vi "TOBECORRECTEDDeviceDiscover.vi"(0 "GenericDevice in":refnum<class "GenericDevice.lvclass">, 5 "error in (no error)":errorcluster) -> (14 "GenericDevice out":refnum<class "GenericDevice.lvclass">, 15 "results-JSON string":string, 16 "ID":i32, 17 "returned command":string, 18 "error string (if existing)":string, 19 "error out":errorcluster)   [LabVIEW 2023, in "GenericDevice.lvclass"]
uses:
  GenericDevice.lvclass
  GenericDevice.lvclass/GenericDevice.ctl
  f3c4c4a7-1197-4301-b128-d95ffad61759.vi
  8dcdfc4e-e41c-41c3-8bf5-06d7d5a87ca3.vi
  <vilib>/JDP Science/JSONtext/Variant to JSON Text.vi
  <vilib>/JDP Science/JSONtext/Set Item.vi
  <vilib>/JDP Science/JSONtext/LVClass Serializer/JSONtext LVClass Serializer.lvclass
panel:
  # "Connector Pane"
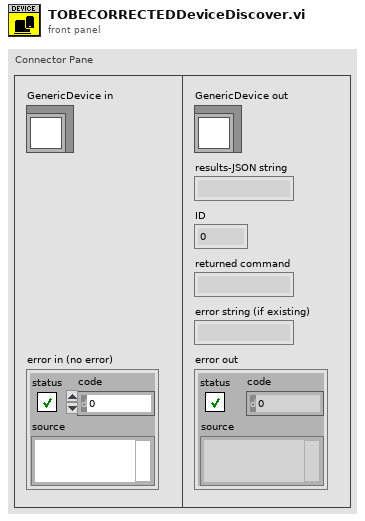
[diagram p1: front panel]
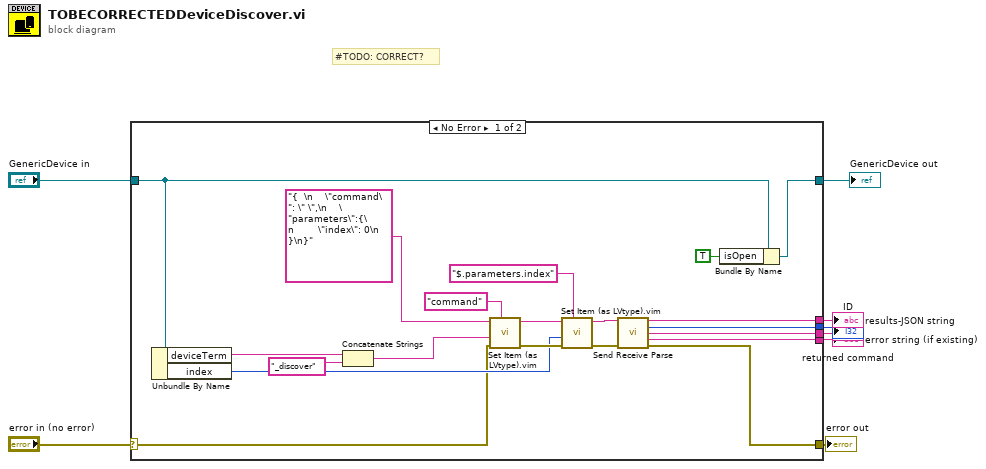
[diagram p0: block diagram]
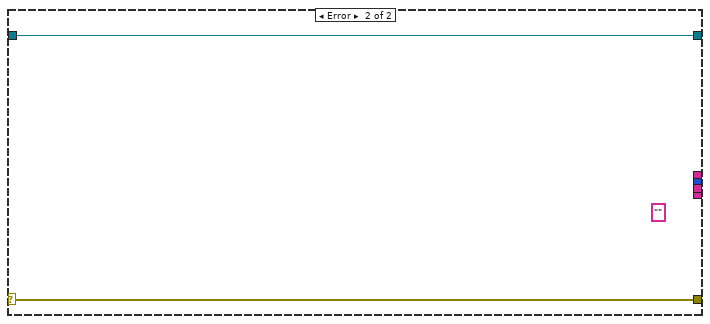
[diagram p2: hidden frame]
diagram:
  # "#TODO: CORRECT?"
  n1 = case shown="No Error" "error in (no error)" {
    selector: "error in (no error)" -> [w19 w30]
    tunnel: [w13 w30] -> w7
    tunnel: [w17 w29] -> w5
    tunnel: "GenericDevice in" -> [w16 w29]
    tunnel: [w12 _] -> w4
    tunnel: [w11 _] -> w3
    tunnel: [w10 _] -> w1
    tunnel: [w9 _] -> w2
    frame No Error {
      n2 = Unbundle By Name(w16) -> ("deviceTerm"=w24:string, "index"=w20:i32)
      n3 = Concatenate Strings(w24, "_discover" ("string")) -> (w21:string)
      n4 = call "Set Item (as LVtype).vim"("$Path or Item Name"="command", "error in (no error)"=w19, "Anything"=w21, "JSON"="{  \n    \"command\": \" \",\n    \"parameters\":{\n        \"index\": 0\n    }\n}") -> ("error out"=w26:errorcluster, "<JSON>"=w27:string)  [unwired: 4 in, 1 out]
      n5 = call "Set Item (as LVtype).vim"("$Path or Item Name"="$.parameters.index", "error in (no error)"=w26, "Anything"=w20, "JSON"=w27) -> ("error out"=w14:errorcluster, "<JSON>"=w15:string)  [unwired: 4 in, 1 out]
      n6 = call "Send Receive Parse.vi"("<JSON>"=w15, "error in"=w14) -> ("results-JSON string"=w12:string, "ID"=w11:i32, "returned command"=w9:string, "error string (if existing)"=w10:string, "error out"=w13:errorcluster)  [unwired: 9 in]
      n7 = Bundle By Name(cluster=w16, "isOpen"=TRUE) -> (w17:refnum<class "GenericDevice.lvclass">)
    }
    frame Error {
      (unwired) "" ("<JSON>")
    }
  }
  "error out" <- w7
  "GenericDevice out" <- w5
  "results-JSON string" <- w4
  "ID" <- w3
  "returned command" <- w2
  "error string (if existing)" <- w1
